vi "shutdown.vi"(8 "error in":errorcluster, 9 "Boiler Simulation Controls":refnum<vi>, 10 "Boiler Controls":refnum<vi>, 11 "Boiler Status Indicators":refnum<vi>) -> (0 "error out":errorcluster, 3 "elapsedTime":dbl)   [LabVIEW 2024]
uses:
  Controls/Boiler Simulation Controls.ctl
  Controls/Boiler Status Indicators.ctl
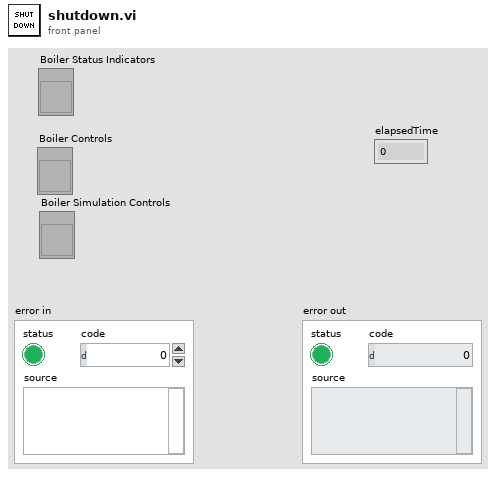
[diagram p1: front panel]
types:
  T1 = typedef "Boiler Status Indicators.ctl" = cluster{"Status":string, "Primary Fan":bool, "Natural Gas Valve":bool, "Pilot":bool, "Fuel Valve":bool, "Forced Draft Fan":bool, "Time Count":dbl}
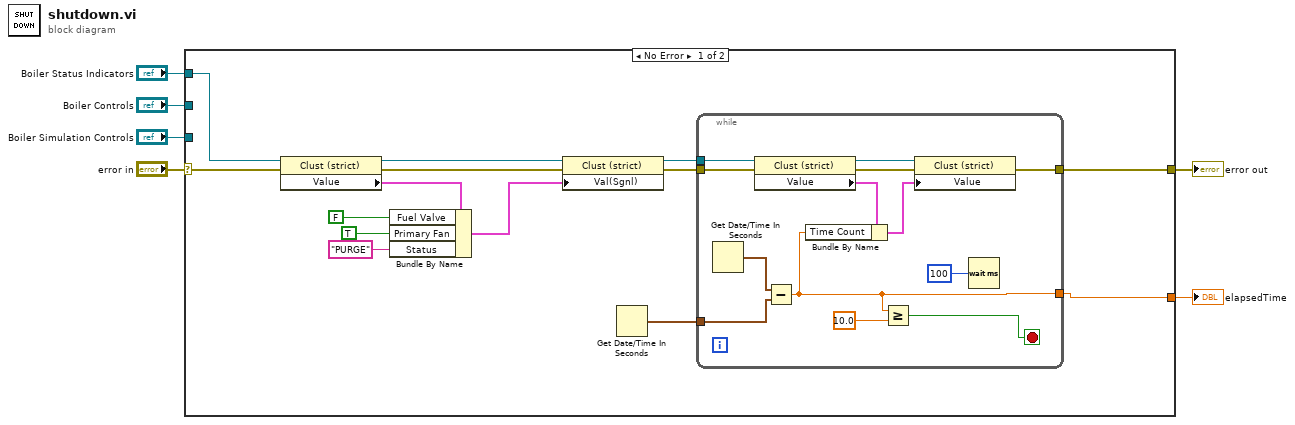
[diagram p0: block diagram]
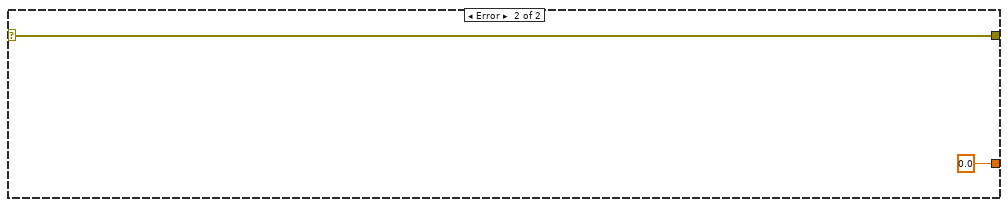
[diagram p2: hidden frame]
diagram:
  n1 = case shown="No Error" "error in" {
    selector: "error in" -> [w20 w35]
    tunnel: [w8 w35] -> w5
    tunnel: "Boiler Status Indicators" -> [w14 _]
    tunnel: "Boiler Controls" -> [_ _]
    tunnel: "Boiler Simulation Controls" -> [_ _]
    tunnel: [w7 0.0] -> w1
    frame No Error {
      n2 = property class="Clust (strict)"(reference=w14, error in=w20) -> (reference out=w17:refnum<vi>, error out=w16:errorcluster, "Value"=w19:T1)
      n3 = Bundle By Name(cluster=w19, "Fuel Valve"=FALSE ("Forced Draft Fan"), "Primary Fan"=TRUE, "Status"="PURGE") -> (w18:T1)
      n4 = property class="Clust (strict)"(reference=w17, error in=w16, "Val(Sgnl)"=w18) -> (reference out=w11:refnum<vi>, error out=w10:errorcluster)
      n5 = Get Date/Time In Seconds() -> (seconds since 1Jan1904=w9:timestamp)
      n6 = while {
        tunnel: w11 -> [w29]
        tunnel: w10 -> [w28]
        tunnel: [w27] -> w8
        tunnel: w9 -> [w25]
        tunnel: [w21] -> w7
        stop <- w23 stop-if-true
        n7 = Get Date/Time In Seconds() -> (seconds since 1Jan1904=w26:timestamp)
        n8 = property class="Clust (strict)"(reference=w29, error in=w28) -> (reference out=w30:refnum<vi>, error out=w31:errorcluster, "Value"=w32:T1)
        n9 = Subtract(x=w26, y=w25) -> (x-y=w21:dbl)
        n10 = Bundle By Name(cluster=w32, "Time Count"=w21) -> (w33:T1)
        n11 = Greater Or Equal?(x=w21, y=10.0) -> (x >= y?=w23:bool)
        n12 = property class="Clust (strict)"(reference=w30, error in=w31, "Value"=w33) -> (error out=w27:errorcluster)  [unwired: 1 out]
        n13 = Wait (ms)(milliseconds to wait=u32 100) -> ()  [unwired: 1 out]
      }
    }
    frame Error {
    }
  }
  "error out" <- w5
  "elapsedTime" <- w1
